vi "Choreo_TrajectoryCacheSwerve_Clear.vi"(8 "error in (no error)":errorcluster) -> (0 "error out":errorcluster)   [LabVIEW 2019, in "ChoreoLib.lvlib"]
doc: "Constructs a SwerveSample with the specified parameters.\n\n */\n\nInputs: \n - t - double - The timestamp of this sample, relative to the beginning of the trajectory.\n - x - double - The X position of the sample in meters.\n - y - double - The Y position of the sample in meters.\n - heading - double - The heading of the sample in radians, with 0 being in the +X direction.\n - vx - double - The velocity of the sample in the X direction in m/s.\n - vy - double - The velocity of the sample in the Y direction in m/s.\n - omega - double - The angular velocity of the sample in rad/s.\n - ax - double - The acceleration of the sample in the X direction in m/s².\n - ay - double - The acceleration of the sample in the Y direction in m/s².\n - alpha - double - The angular acceleration of the sample in rad/s².\n - moduleForcesX - double array - The force on each swerve module in the X direction in Newtons. Module forces appear in the following order: [FL, FR, BL, BR].\n - moduleForcesY - double array - The force on each swerve module in the Y direction in Newtons. Module forces appear in the following order: [FL, FR, BL, BR].\n\nOutputs:\n - ChoreoSwerveSample - cluster - Cluster containing sample data"
uses:
  ChoreoLib.lvlib
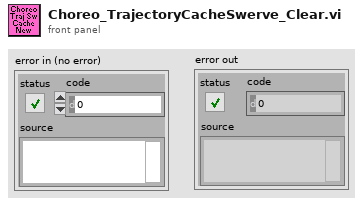
[diagram p1: front panel]
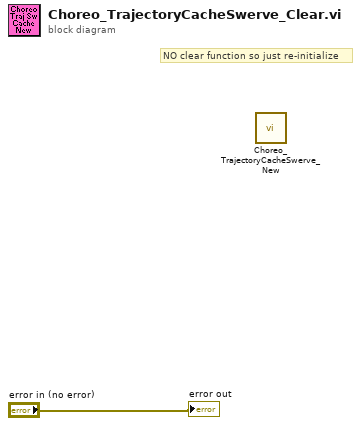
[diagram p0: block diagram]
diagram:
  # "NO clear function so just re-initialize"
  n1 = call "Choreo_TrajectoryCacheSwerve_New.vi"() -> ()  [unwired: 12 in]
  "error out" <- "error in (no error)"
